vi "Add Channel to Objects.vi"(8 "error in":errorcluster, 9 "success":bool, 10 "line item in":T1, 11 "Objects in":T4) -> (0 "error out":errorcluster)   [LabVIEW 2013, in "Scan Engine editor node.lvclass"]
uses:
  Scan Engine editor node.lvclass
  <vilib>/NI/DCAF Table API/Table Manager/object ref.ctl
  <vilib>/NI/DCAF/Tag Editor Core/Configuration Editor/Classes/Engine Parent/Engine Parent Editor Node.lvclass
  <vilib>/NI/DCAF/Tag Editor Core/Configuration Editor/Classes/Module editor node/module editor node.lvclass
  Mappings.ctl
  <vilib>/NI/Tag Bus Module Framework/channel/TBM channel.lvclass
  module/configuration/Line.ctl
  Map.ctl
  module/configuration/Scan Engine configuration.lvclass
  <vilib>/NI/Configuration Framework/serializable configuration/NISE_CEF_serializable configuration.lvclass/NISE_CEF_serializable configuration.ctl
  <vilib>/Utility/LVClass/Get LV Class Name.vi
  <vilib>/NI/Configuration Framework/error generator/NISE_error generator.vi
  <vilib>/NI/Configuration Framework/serializable configuration/NISE_CEF_serializable configuration.lvclass
  <vilib>/NI/DCAF Table API/Table Manager/Table Manager.lvclass
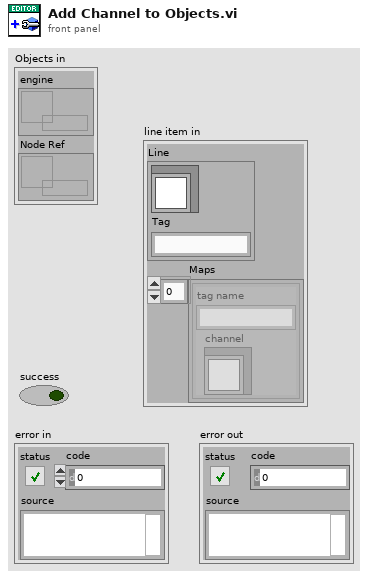
[diagram p1: front panel]
types:
  T1 = typedef "Scan Engine editor node.lvclass/Mappings.ctl" = cluster{"Line":T2, "Maps":T3[]}
  T2 = typedef "Scan Engine configuration.lvclass/Line.ctl" = cluster{"channel":refnum<class "TBM channel.lvclass">, "Tag":string}
  T3 = typedef "Scan Engine editor node.lvclass/Map.ctl" = cluster{"channel":refnum<class "TBM channel.lvclass">, "tag name":string}
  T4 = typedef "Table Manager.lvlib/Table Manager.lvclass/object ref.ctl" = cluster{"engine":refnum<data-value>, "Node Ref":refnum<data-value>}
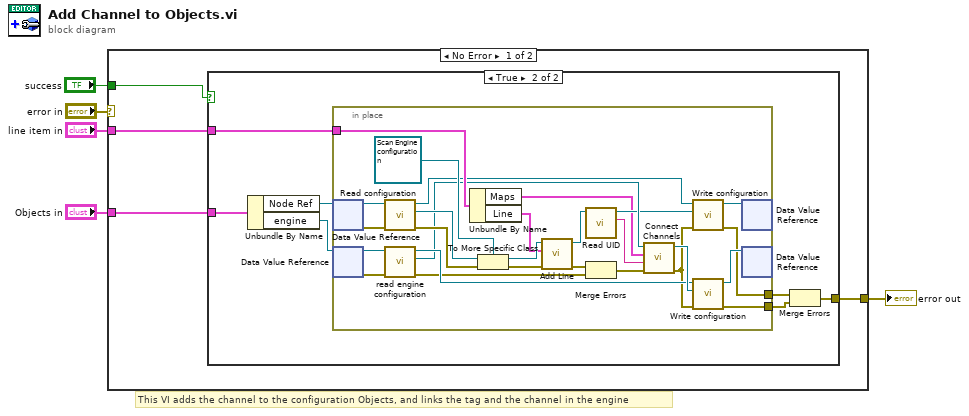
[diagram p0: block diagram]
diagram:
  # "This VI adds the channel to the configuration Objects, and links the tag and the channel in the engine"
  n1 = case shown="No Error" "error in" {
    selector: "error in" -> [_ w44]
    tunnel: "Objects in" -> [w9 _]
    tunnel: "line item in" -> [w8 _]
    tunnel: "success" -> [w7 _]
    tunnel: [w6 w44] -> w1
    frame No Error {
      n2 = case shown="True" w7 {
        tunnel: [_ w14] -> w6
        tunnel: w8 -> [_ w16]
        tunnel: w9 -> [_ w15]
        frame False {
        }
        frame True {
          n3 = Unbundle By Name(w15) -> ("Node Ref"=w13:refnum<data-value>, "engine"=w12:refnum<data-value>)
          n4 = in-place {
            in-place-border: w16 -> [w43]
            in-place-border: [w30] -> w11
            in-place-border: [w28] -> w10
            n5 = in-place-dvr #1(w13) -> (w37:refnum<class "module editor node.lvclass">, w29:errorcluster)
            n6 = in-place-dvr #2(w12) -> (w27:refnum<class "Engine Parent Editor Node.lvclass">, w26:errorcluster)
            n7 = call-dynamic "Read configuration.vi"("error in"=w29, "NISE_CEF_serializable node in"=w37) -> ("error out"=w31:errorcluster, "configuration"=w32:refnum<class "NISE_CEF_serializable configuration.lvclass">, "NISE_CEF_serializable node out"=w36:refnum<class "module editor node.lvclass">)  [unwired: 7 in]
            n8 = call <vilib>:"read engine configuration.vi"("error in"=w26, "Engine Parent Editor Node in"=w27) -> ("error out"=w23:errorcluster, "engine configuration"=w24:refnum<class "engine configuration.lvclass">, "Engine Parent Editor Node out"=w25:refnum<class "Engine Parent Editor Node.lvclass">)  [unwired: 7 in]
            n9 = Unbundle By Name(w43) -> ("Maps"=w19:T3[], "Line"=w18:T2)
            n10 = To More Specific Class(target class=refnum<class "Scan Engine configuration.lvclass"> refnum ("tag bus configurable plugin module configuration in"), reference=w32, error in=w31) -> (specific class reference=w41:refnum<class "Scan Engine configuration.lvclass">, error out=w40:errorcluster)
            n11 = call "Add Line.vi"("error in"=w40, "Line"=w18, "Scan Engine configuration in"=w41) -> ("error out"=w39:errorcluster, "Scan Engine configuration out"=w22:refnum<class "Scan Engine configuration.lvclass">)  [unwired: 7 in]
            n12 = call <vilib>:"Read UID.vi"("configuration in"=w22) -> ("instance id"=w21:string, "configuration out"=w20:refnum<class "Scan Engine configuration.lvclass">)  [unwired: 8 in, 1 out]
            n13 = Merge Errors(w39, w23) -> (w38:errorcluster)
            n14 = call "Connect Channels.vi"("error in (no error)"=w38, "instance id"=w21, "Maps"=w19, "engine configuration in"=w24) -> ("error out"=w17:errorcluster, "engine configuration out"=w33:refnum<class "engine configuration.lvclass">)  [unwired: 6 in]
            n15 = call-dynamic "Write configuration.vi"("error in"=w17, "configuration"=w20, "NISE_CEF_serializable node in"=w36) -> ("error out"=w28:errorcluster, "NISE_CEF_serializable node out"=w35:refnum<class "module editor node.lvclass">)  [unwired: 7 in]
            n16 = call-dynamic "Write configuration.vi"("error in"=w17, "configuration"=w33, "NISE_CEF_serializable node in"=w25) -> ("error out"=w30:errorcluster, "NISE_CEF_serializable node out"=w34:refnum<class "Engine Parent Editor Node.lvclass">)  [unwired: 7 in]
            n17 = in-place-dvr #1(w35) -> ()  [unwired: 2 out]
            n18 = in-place-dvr #2(w34) -> ()  [unwired: 2 out]
          }
          n19 = Merge Errors(w10, w11) -> (w14:errorcluster)
        }
      }
    }
    frame Error {
    }
  }
  "error out" <- w1
